vi "Do Request.vi"(7 "Processing In":refnum<class "Processing.lvclass">, 11 "TestCSRFController in":refnum<class "TestCSRFController.lvclass">) -> (0 "error out":errorcluster, 5 "Processing":refnum<class "Processing.lvclass">)   [LabVIEW 2020, in "TestCSRFController.lvclass"]
uses:
  TestCSRFController.lvclass
  <vilib>/IlluminatedG/IG HTTP Server/HTTP Server/Processing/Processing.lvclass
  <vilib>/IlluminatedG/IG HTTP Server/HTTP Server/Processing/Processing.lvclass/Processing.ctl
  <vilib>/IlluminatedG/IG HTTP Utils/HTTP Utils/Request/Get Target URI.vi
  <vilib>/IlluminatedG/lv-stream/URI/Get Path.vi
  <vilib>/IlluminatedG/IG HTTP Server/HTTP Server/Session/Session.lvclass
  <vilib>/IlluminatedG/IG HTTP Utils/HTTP Utils/Response/Response.lvclass
  <vilib>/IlluminatedG/IG HTTP Utils/HTTP Utils/Request/Request.lvclass
  <vilib>/IlluminatedG/IG HTTP Utils/HTTP Utils/FormField/FormField.lvclass
  <vilib>/IlluminatedG/IG HTTP Server/HTTP Server/HTTP Server.lvlib
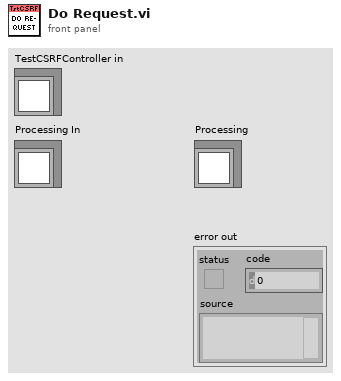
[diagram p1: front panel]
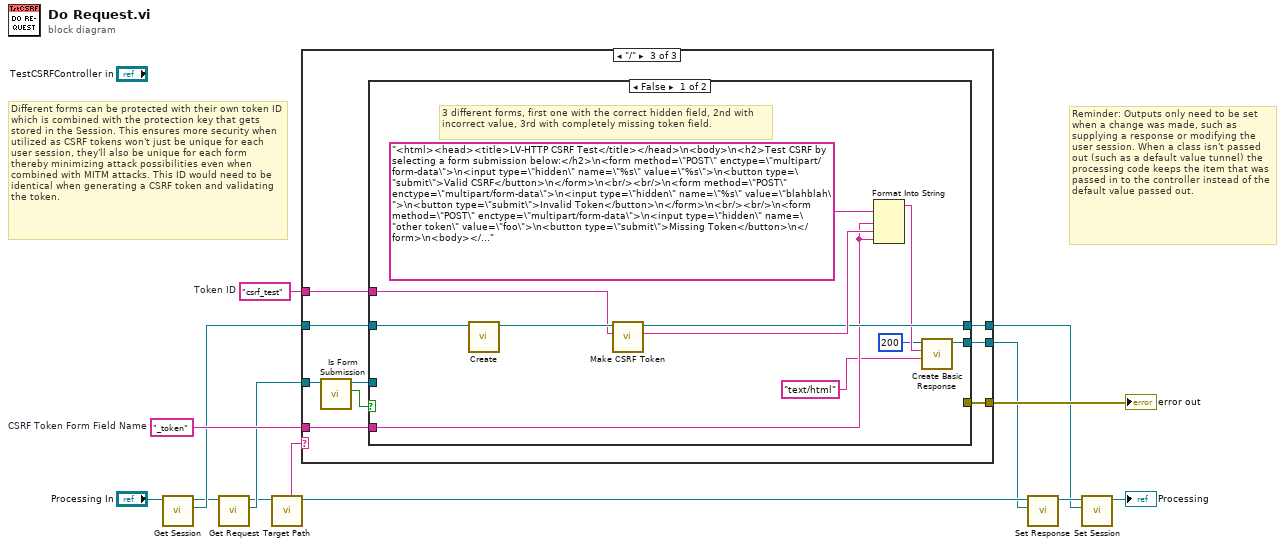
[diagram p0: block diagram]
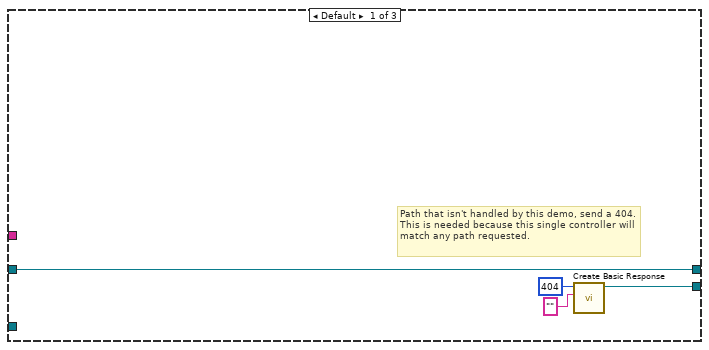
[diagram p2: hidden frame]
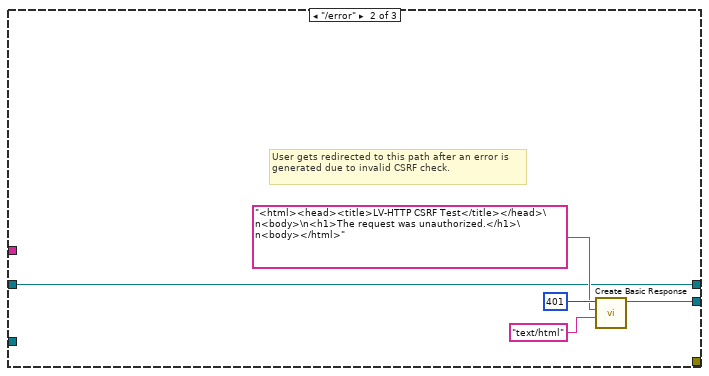
[diagram p3: hidden frame]
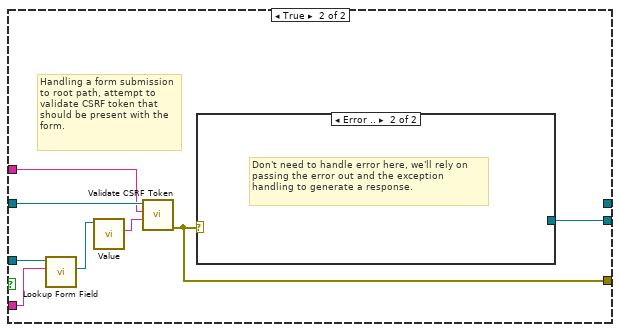
[diagram p4: hidden frame]
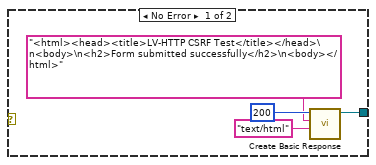
[diagram p5: hidden frame]
diagram:
  w13 = "_token"  # CSRF Token Form Field Name
  w14 = "csrf_test"  # Token ID
  # "Different forms can be protected with their own token ID which is combined with the protection key that gets stored in the Session. This ensures more security when utilized as CSRF tokens won't just be unique for each user session, they'll also be unique for each form thereby minimizing attack possibilities even when combined with MITM attacks. This ID would need to be identical when generating a CSRF token and validating the token."
  # "Reminder: Outputs only need to be set when a change was made, such as supplying a response or modifying the user session. When a class isn't passed out (such as a default value tunnel) the processing code keeps the item that was passed in to the controller instead of the default value passed out."
  n1 = call <vilib>:"Get Session.vi"("Processing in"="Processing In") -> ("Session"=w9:refnum<class "Session.lvclass">, "Processing out"=w8:refnum<class "Processing.lvclass">)  [unwired: 9 in]
  n2 = call <vilib>:"Get Request.vi"("Processing in"=w8) -> ("Request"=w7:refnum<class "Request.lvclass">, "Processing out"=w6:refnum<class "Processing.lvclass">)  [unwired: 9 in]
  n3 = call <vilib>:"Target Path.vi"("Processing in"=w6) -> ("Processing out"=w5:refnum<class "Processing.lvclass">, "Target Path"=w11:string)  [unwired: 9 in]
  n4 = case shown="\"/\"" w11 {
    tunnel: w9 -> [w15 w20 w29]
    tunnel: w7 -> [_ _ w27]
    tunnel: [w16 w23 w32] -> w4
    tunnel: [w15 w20 w31] -> w2
    tunnel: w14 -> [_ _ w28]
    tunnel: w13 -> [_ _ w30]
    tunnel: [_ _ w24] -> w12
    frame Default {
      # "Path that isn't handled by this demo, send a 404. This is needed because this single controller will match any path requested."
      n5 = call <vilib>:"Create Basic Response.vi"("Payload"="", "Status Code"=u16 404) -> ("Response out"=w16:refnum<class "Response.lvclass">)  [unwired: 8 in, 1 out]
    }
    frame "/error" {
      # "User gets redirected to this path after an error is generated due to invalid CSRF check."
      n6 = call <vilib>:"Create Basic Response.vi"("Content-Type (text/plain)"="text/html", "Payload"="<html><head><title>LV-HTTP CSRF Test</title></head>\n<body>\n<h1>The request was unauthorized.</h1>\n<body></html>", "Status Code"=u16 401) -> ("Response out"=w23:refnum<class "Response.lvclass">)  [unwired: 7 in, 1 out]
    }
    frame "/" {
      n7 = call <vilib>:"Is Form Submission.vi"("Request in"=w27) -> ("Is Form Submission?"=w26:bool, "Request out"=w25:refnum<class "Request.lvclass">)  [unwired: 8 in, 1 out]
      n8 = case shown="False" w26 {
        tunnel: [w43 w47] -> w32
        tunnel: [w40 _] -> w31
        tunnel: w30 -> [w39 w46]
        tunnel: w29 -> [w33 w49]
        tunnel: w28 -> [w34 w45]
        tunnel: w25 -> [_ w48]
        tunnel: [_ w44] -> w24
        frame False {
          # "3 different forms, first one with the correct hidden field, 2nd with incorrect value, 3rd with completely missing token field."
          n9 = call <vilib>:"Create.vi"("Session in"=w33) -> ("Session out"=w35:refnum<class "Session.lvclass">)  [unwired: 9 in, 1 out]
          n10 = call <vilib>:"Make CSRF Token.vi"("Token ID"=w34, "Session In"=w35) -> ("Token"=w41:string, "Session"=w40:refnum<class "Session.lvclass">)  [unwired: 7 in, 1 out]
          n11 = Format Into String(format string="<html><head><title>LV-HTTP CSRF Test</title></head>\n<body>\n<h2>Test CSRF by selecting a form submission below:</h2>\n<form method=\"POST\" enctype=\"multipart/form-data\">\n<input type=\"hidden\" name=\"%s\" value=\"%s\">\n<button type=\"submit\">Valid CSRF</button>\n</form>\n<br/><br/>\n<form method=\"POST\" enctype=\"multipart/form-data\">\n<input type=\"hidden\" name=\"%s\" value=\"blahblah\">\n<button type=\"submit\">Invalid Token</button>\n</form>\n<br/><br/>\n<form method=\"POST\" enctype=\"multipart/form-data\">\n<input type=\"hidden\" name=\"other token\" value=\"foo\">\n<button type=\"submit\">Missing Token</button>\n</form>\n<body></html>", w39, w41, w39) -> (resulting string=w38:string)  [unwired: 2 in, 1 out]
          n12 = call <vilib>:"Create Basic Response.vi"("Content-Type (text/plain)"="text/html", "Payload"=w38, "Status Code"=u16 200) -> ("Response out"=w43:refnum<class "Response.lvclass">)  [unwired: 7 in, 1 out]
        }
        frame True {
          # "Handling a form submission to root path, attempt to validate CSRF token that should be present with the form."
          n13 = call <vilib>:"Lookup Form Field.vi"("Name"=w46, "Request in"=w48) -> ("Field"=w51:refnum<class "FormField.lvclass">)  [unwired: 6 in, 3 out]
          n14 = call <vilib>:"Value.vi"("FormField in"=w51) -> ("Value"=w50:string)  [unwired: 8 in, 2 out]
          n15 = call <vilib>:"Validate CSRF Token.vi"("Token"=w50, "Token ID"=w45, "Session In"=w49) -> ("error out"=w44:errorcluster)  [unwired: 7 in, 1 out]
          n16 = case shown="Error .." w44 {
            tunnel: [w55 _] -> w47
            frame No Error {
              n17 = call <vilib>:"Create Basic Response.vi"("Content-Type (text/plain)"="text/html", "Payload"="<html><head><title>LV-HTTP CSRF Test</title></head>\n<body>\n<h2>Form submitted successfully</h2>\n<body></html>", "Status Code"=u16 200) -> ("Response out"=w55:refnum<class "Response.lvclass">)  [unwired: 7 in, 1 out]
            }
            frame Error {
              # "Don't need to handle error here, we'll rely on passing the error out and the exception handling to generate a response."
            }
          }
        }
      }
    }
  }
  "error out" <- w12
  n18 = call <vilib>:"Set Response.vi"("Response"=w4, "Processing in"=w5) -> ("Processing out"=w3:refnum<class "Processing.lvclass">)  [unwired: 9 in]
  n19 = call <vilib>:"Set Session.vi"("Session"=w2, "Processing in"=w3) -> ("Processing out"=→"Processing":refnum<class "Processing.lvclass">)  [unwired: 9 in]
